vi "DACmapping.vi"(8 "error in (no error)":errorcluster, 11 "DAC_TH":u32) -> (0 "error out":errorcluster, 2 "COMB DEC":i64=255)   [LabVIEW 2012]
panel:
  out "?":bool[](array[boolean])=[TRUE, TRUE, TRUE, TRUE, TRUE, TRUE, TRUE, TRUE, FALSE, FALSE, FALSE, FALSE, FALSE, FALSE, FALSE, FALSE, FALSE, FALSE, FALSE, FALSE, FALSE, FALSE, FALSE, FALSE, FALSE, FALSE, FALSE, FALSE, FALSE, FALSE, FALSE, FALSE, FALSE, FALSE, FALSE, FALSE, FALSE, FALSE, FALSE, FALSE, FALSE, FALSE, FALSE, FALSE, FALSE, FALSE, FALSE, FALSE, FALSE, FALSE, FALSE, FALSE, FALSE, FALSE, FALSE, FALSE, FALSE, FALSE, FALSE, FALSE, FALSE, FALSE, FALSE, FALSE]
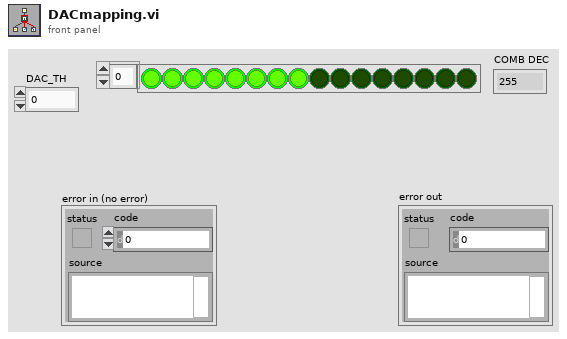
[diagram p1: front panel]
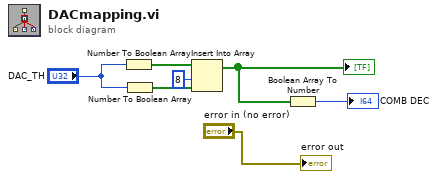
[diagram p0: block diagram]
diagram:
  n1 = Number To Boolean Array(number="DAC_TH") -> (Boolean array=w7:bool[])
  n2 = Number To Boolean Array(number="DAC_TH") -> (Boolean array=w6:bool[])
  n3 = Insert Into Array(array=w7, index=8, new element=w6) -> (w5:bool[])
  "?" <- w5
  n4 = Boolean Array To Number(Boolean array=w5) -> (number=→"COMB DEC":u32)
  "error out" <- "error in (no error)"
